vi "Simple Command Pattern.vi"() -> ()   [LabVIEW 2018]
doc: "Use this template to build a producer/consumer design pattern. Use this template when you need to execute a process, such as data analysis, when a data source, such as a triggered acquisition, produces data at an uneven rate and you need to execute the process when the data becomes available."
uses:
  Action_class/Action.lvclass
  Exit_class/Exit.lvclass
  C:/GitClones/LVOOP DRAFT/Command Pattern/Action_class/Action.lvclass
panel:
  in  "Do Action":bool
  in  "stop":bool
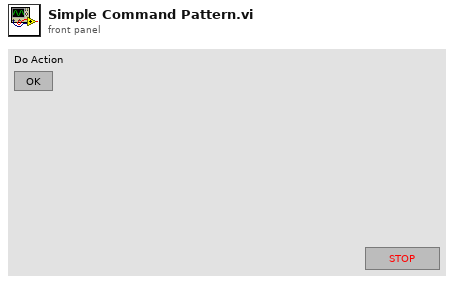
[diagram p1: front panel]
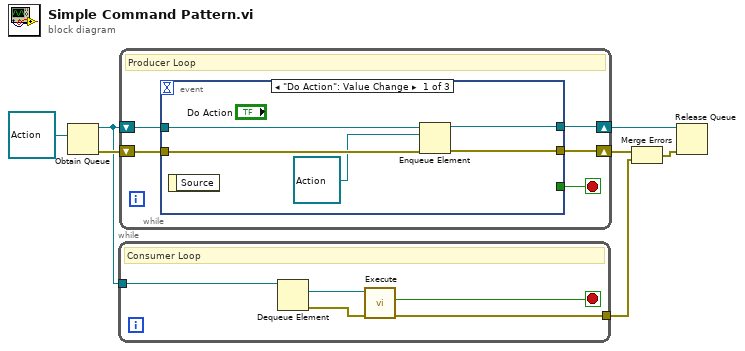
[diagram p0: block diagram]
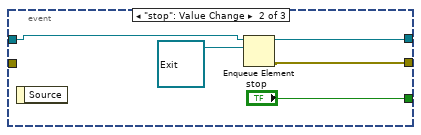
[diagram p2: hidden frame]
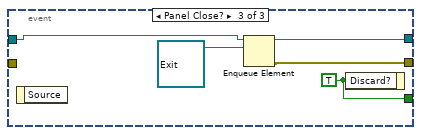
[diagram p3: hidden frame]
diagram:
  n1 = Obtain Queue(element data type=refnum<class "Action.lvclass"> refnum ("Action.lvclass")) -> (queue out=w3:refnum<queue>, error out=w4:errorcluster)  [unwired: 4 in, 1 out]
  n2 = while {
    tunnel: w3 -> [w11]
    tunnel: [w12] -> w1
    stop <- w8 stop-if-true
    # "Consumer Loop"
    n3 = Dequeue Element(queue=w11) -> (element=w10:refnum<class "Action.lvclass">, error out=w9:errorcluster)  [unwired: 2 in, 2 out]
    n4 = call-dynamic "Execute.vi"("error in (no error)"=w9, "Action in"=w10) -> ("error out"=w12:errorcluster, "Exit?"=w8:bool)  [unwired: 7 in, 1 out]
  }
  n5 = while {
    shift-right: [w14] -> w6
    shift-left: w4 -> [w15]
    shift-right: [w16] -> w7
    shift-left: w3 -> [w17]
    stop <- w13 stop-if-true
    # "Producer Loop"
    n6 = event shown="[0] \"Do Action\": Value Change" {
      selector: _ -> [_ _ _]
      dyn-events: _ -> [_ _ _]
      timeout: _ -> [_ _ _]
      tunnel: w17 -> [w22 w26 w32]
      tunnel: [w21 w24 w30] -> w16
      tunnel: w15 -> [w20 _ _]
      tunnel: [w19 w23 w29] -> w14
      tunnel: [_ "stop" w28] -> w13
      event "Do Action": Value Change {
        n7 = event-data() -> ()  [unwired: 1 in, 1 out]
        n8 = Enqueue Element(queue=w22, element=refnum<class "Action.lvclass"> refnum ("Action.lvclass"), error in (no error)=w20) -> (queue out=w21:refnum<queue>, error out=w19:errorcluster)  [unwired: 1 in, 1 out]
      }
      event "stop": Value Change {
        n9 = event-data() -> ()  [unwired: 1 in, 1 out]
        n10 = Enqueue Element(queue=w26, element=refnum<class "Exit.lvclass"> refnum ("Message")) -> (queue out=w24:refnum<queue>, error out=w23:errorcluster)  [unwired: 2 in, 1 out]
      }
      event Panel Close? {
        w28 = TRUE ("Discard?")
        n11 = event-data() -> ()  [unwired: 1 in, 1 out]
        n12 = Enqueue Element(queue=w32, element=refnum<class "Exit.lvclass"> refnum ("Message")) -> (queue out=w30:refnum<queue>, error out=w29:errorcluster)  [unwired: 2 in, 1 out]
        n13 = event-data("Discard?"=w28) -> ()  [unwired: 1 in, 1 out]
      }
    }
  }
  n14 = Merge Errors(w6, w1) -> (w5:errorcluster)
  n15 = Release Queue(queue=w7, error in (no error)=w5) -> ()  [unwired: 1 in, 3 out]
